vi "Rename items.vi"(10 "New Name":string="NewName", 11 "Pattern":string="[TEST]") -> ()   [LabVIEW 2019, in "ProjectItem.lvclass"]
uses:
  ProjectItem.lvclass
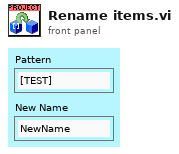
[diagram p1: front panel]
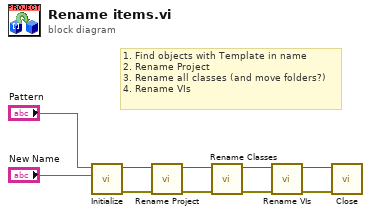
[diagram p0: block diagram]
diagram:
  # "1. Find objects with Template in name\n2. Rename Project\n3. Rename all classes (and move folders?)\n4. Rename VIs"
  n1 = call "Initialize.vi"("New Name"="New Name", "Pattern"="Pattern") -> ("error out"=w10:errorcluster, "ProjectItem out"=w9:refnum<class "ProjectItem.lvclass">)  [unwired: 8 in]
  n2 = call "Rename Project.vi"("error in (no error)"=w10, "ProjectItem in"=w9) -> ("error out"=w5:errorcluster, "ProjectItem out"=w6:refnum<class "ProjectItem.lvclass">)  [unwired: 8 in]
  n3 = call "Rename Classes.vi"("error in (no error)"=w5, "ProjectItem in"=w6) -> ("error out"=w3:errorcluster, "ProjectItem out"=w4:refnum<class "ProjectItem.lvclass">)  [unwired: 8 in]
  n4 = call "Rename VIs.vi"("error in (no error)"=w3, "ProjectItem in"=w4) -> ("error out"=w1:errorcluster, "ProjectItem out"=w2:refnum<class "ProjectItem.lvclass">)  [unwired: 8 in]
  n5 = call "Close.vi"("error in (no error)"=w1, "ProjectItem in"=w2) -> ()  [unwired: 8 in, 2 out]
